vi "Read SSH Client.vi"(8 "error in (no error)":errorcluster, 11 "session in":refnum<class "Session.lvclass">) -> (0 "error out":errorcluster, 2 "NI_SSH.lvlib:SSH Client":refnum<class "Generic Client.lvclass">, 3 "session out":refnum<class "Session.lvclass">)   [LabVIEW 2020, in "NI_SFTP.lvlib" / "Session.lvclass"]
uses:
  <vilib>/net/SFTP/Session/Session.lvclass
  <vilib>/net/SSH/Client/Generic/Generic Client.lvclass
  <vilib>/net/SFTP/Session/Session.lvclass/Session.ctl
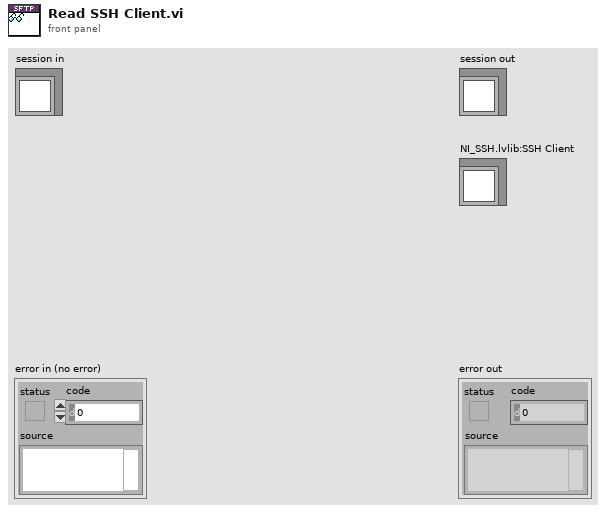
[diagram p1: front panel]
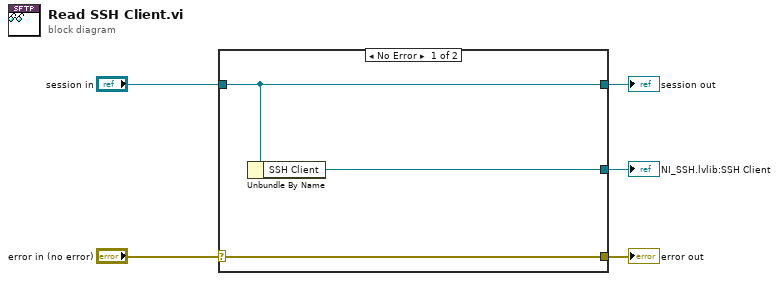
[diagram p0: block diagram]
diagram:
  n1 = case shown="No Error" "error in (no error)" {
    selector: "error in (no error)" -> [w8 w9]
    tunnel: [w8 w9] -> w4
    tunnel: [w7 w10] -> w2
    tunnel: "session in" -> [w7 w10]
    tunnel: [w6 _] -> w1
    frame No Error {
      n2 = Unbundle By Name(w7) -> ("SSH Client"=w6:refnum<class "Generic Client.lvclass">)
    }
    frame Error {
    }
  }
  "error out" <- w4
  "session out" <- w2
  "NI_SSH.lvlib:SSH Client" <- w1
